vi "INV B - Current Sense Test.vi"(8 "error in (no error)":errorcluster, 10 "Message IN":string, 11 "Board Selector":T1) -> (0 "error out":errorcluster, 1 "Result (bool)":bool, 2 "Message OUT":string, 3 "VISA OUT":refnum<visa-resource-name>, 5 "Sense W":dbl, 7 "Sense V":dbl, 9 "Sense U":dbl)   [LabVIEW 2022 SP3]
uses:
  Serial Board Com/Board Select.ctl
  Serial Board Com/ADCSelector BB.ctl
  Serial Board Com/ADCSelector GB.ctl
  HMP4000 Communication/HMP4040_ChannelControl.ctl
panel:
  out "INVA_ISENSE_W":bool
  out "INVA_ISENSE_V":bool
  out "INVA_ISENSE_U":bool
  out "Result (color)":u32(colorbox)
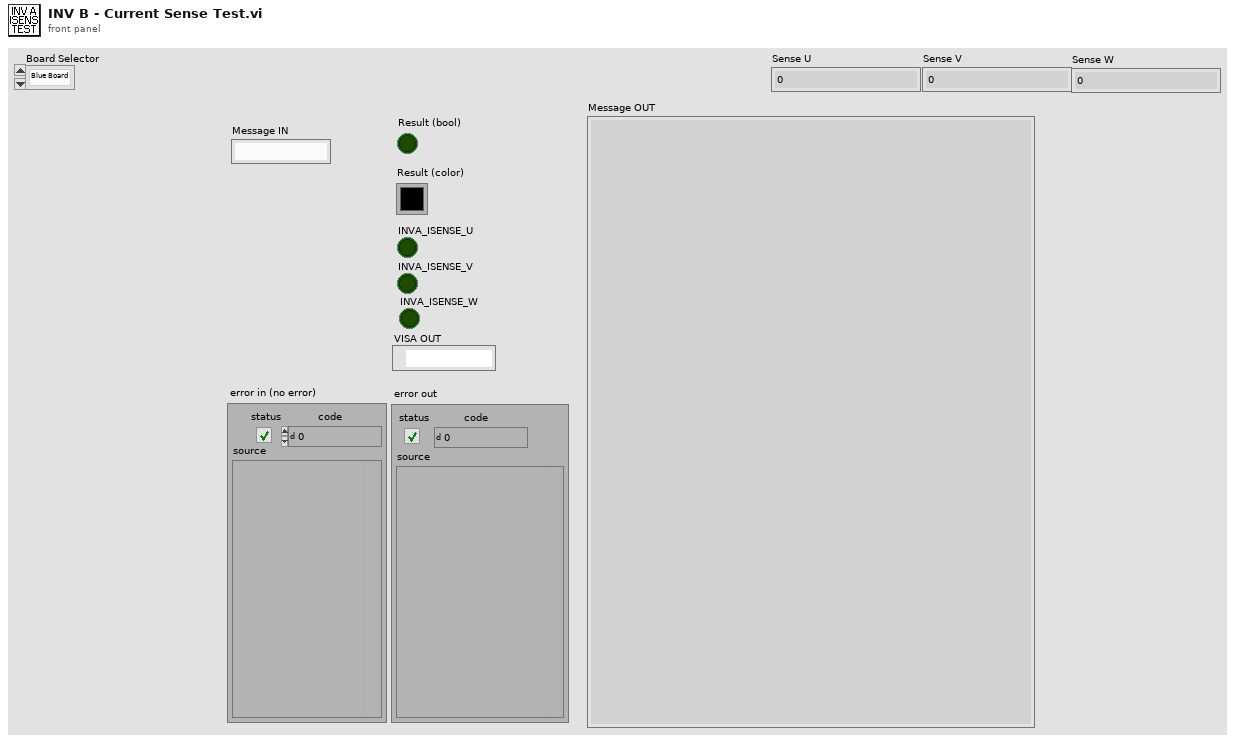
[diagram p1: front panel]
types:
  T1 = typedef "Board Select.ctl" = enum16{"Blue Board", "Green Board"}
  T2 = typedef "HMP4040_ChannelControl.ctl" = cluster{"CH1 Voltage":dbl, "CH1 Current":dbl, "CH1 Output":bool, "CH2 Voltage":dbl, "CH2 Current":dbl, "CH2 Output":bool, "CH3 Voltage":dbl, "CH3 Current":dbl, "CH3 Output":bool, "CH4 Voltage":dbl, "CH4 Current":dbl, "CH4 Output":bool, "Master Output":bool}
  T3 = typedef "ADCSelector GB.ctl" = enum16{"INVA_ISENSE_U", "INVA_ISENSE_V", "INVA_ISENSE_W", "INVA_UDC", "INVA_TEMP", "HB_ISENSE", "AUX_ISENSE_U", "AUX_ISENSE_V", "AUX_ISENSE_W", "VLINE_AB", "VLINE_BC", "VLINE_CA", "REF_1P5V", "VSENSE_POS_24V", "VSENSE_POS_5V", "VSENSE_NEG_15V", "TEST_POINT", "INVB_ISENSE_U", "INVB_ISENSE_V", "INVB_ISENSE_W", "INVB_UDC", "INVB_TEMP", "HB_TEMP", "AUXA_TEMP", "AUXB_TEMP", "AUXC_TEMP", "VOUT_AB", "VOUT_BC", "VOUT_CA", "REF_2P5V", "VSENSE_POS_15V", "VSENSE_POS_3P3V", "NET_ANALYZER"}
  T4 = typedef "ADCSelector BB.ctl" = enum16{"INVA_ISENSE_U", "INVA_ISENSE_V", "INVA_ISENSE_W", "INVA_UDC", "INVA_TEMP", "HB_TEMP", "AUXB_TEMP", "VLINE_AB", "VLINE_BC", "VLINE_CA", "VSENSE_POS_24V", "VSENSE_POS_5V", "VSENSE_NEG_15V", "INVB_ISENSE_U", "INV_B_ISENSEV", "INVB_ISENSE_W", "INVB_UDC", "INVB_TEMP", "AUXA_TEMP", "AUXC_TEMP", "VOUT_AB", "VOUT_BC", "VOUT_CA", "VSENSE_POS_15V", "VSENSE_POS_3P3V", "TEST_POINT"}
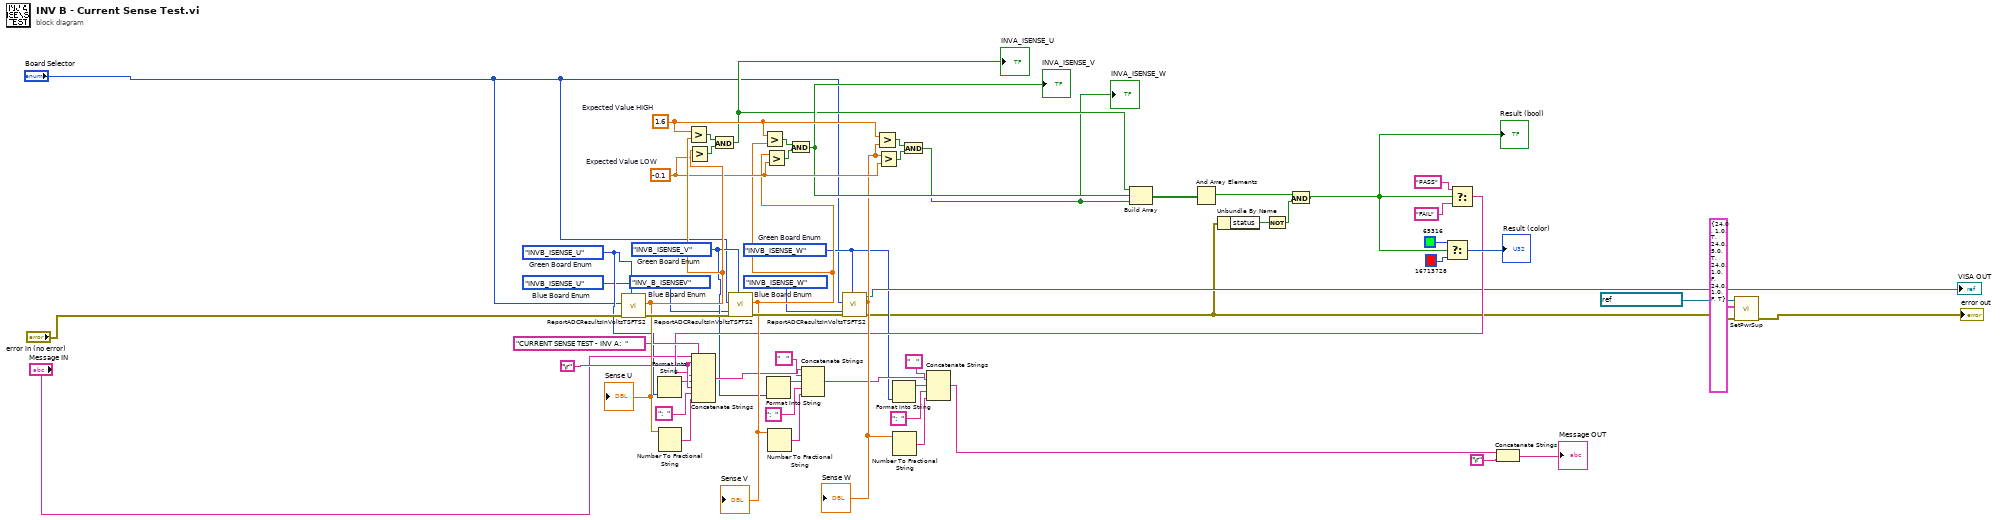
[diagram p0: block diagram]
diagram:
  w9 = ADCSelector_GB."INVB_ISENSE_W"  # Green Board Enum
  w10 = ADCSelector_GB."INVB_ISENSE_V"  # Green Board Enum
  w11 = ADCSelector_GB."INVB_ISENSE_U"  # Green Board Enum
  w16 = "\r"
  w33 = -0.1  # Expected Value LOW
  w32 = 1.6  # Expected Value HIGH
  w1 = ADCSelector_BB."INVB_ISENSE_W"  # Blue Board Enum
  w2 = ADCSelector_BB."INV_B_ISENSEV"  # Blue Board Enum
  w3 = ADCSelector_BB."INVB_ISENSE_U"  # Blue Board Enum
  n1 = call "ReportADCResultsInVoltsTSFTS2.vi"("Blue Board Enum"=w3, "Green Board Enum"=w11, "error in (no error)"="error in (no error)", "Board Selector"="Board Selector") -> ("error out"=w50:errorcluster, "Result"=w40:dbl)  [unwired: 4 in, 2 out]
  "Sense U" <- w40
  n2 = Format Into String(w11) -> (resulting string=w17:string)  [unwired: 3 in, 1 out]
  n3 = Number To Fractional String(number=w40) -> (F-format string=w19:string)  [unwired: 3 in]
  n4 = Greater?(x=w32, y=w40) -> (0:w39:bool)
  n5 = Greater?(x=w40, y=w33) -> (0:w38:bool)
  n6 = And(x=w39, y=w38) -> (x .and. y?=w30:bool)
  "INVA_ISENSE_U" <- w30
  n7 = call "ReportADCResultsInVoltsTSFTS2.vi"("Blue Board Enum"=w2, "Green Board Enum"=w10, "error in (no error)"=w50, "Board Selector"="Board Selector") -> ("error out"=w49:errorcluster, "Result"=w29:dbl)  [unwired: 4 in, 2 out]
  "Sense V" <- w29
  n8 = Greater?(x=w32, y=w29) -> (0:w36:bool)
  n9 = Greater?(x=w29, y=w33) -> (0:w37:bool)
  n10 = Format Into String(w10) -> (resulting string=w46:string)  [unwired: 3 in, 1 out]
  n11 = Number To Fractional String(number=w29) -> (F-format string=w47:string)  [unwired: 3 in]
  n12 = And(x=w36, y=w37) -> (x .and. y?=w31:bool)
  "INVA_ISENSE_V" <- w31
  n13 = call "ReportADCResultsInVoltsTSFTS2.vi"("Blue Board Enum"=w1, "Green Board Enum"=w9, "error in (no error)"=w49, "Board Selector"="Board Selector") -> ("error out"=w8:errorcluster, "Result"=w28:dbl, "VISA Refnum out"=→"VISA OUT":refnum<visa-resource-name>)  [unwired: 4 in, 1 out]
  "Sense W" <- w28
  n14 = Greater?(x=w32, y=w28) -> (0:w35:bool)
  n15 = Greater?(x=w28, y=w33) -> (0:w34:bool)
  n16 = Format Into String(w9) -> (resulting string=w45:string)  [unwired: 3 in, 1 out]
  n17 = Number To Fractional String(number=w28) -> (F-format string=w44:string)  [unwired: 3 in]
  n18 = And(x=w35, y=w34) -> (x .and. y?=w27:bool)
  "INVA_ISENSE_W" <- w27
  n19 = Build Array(w30, w31, w27) -> (w42:bool[])
  n20 = And Array Elements(Boolean array=w42) -> (logical AND=w53:bool)
  n21 = Unbundle By Name(w8) -> ("status"=w41:bool)
  n22 = Not(x=w41) -> (.not. x?=w52:bool)
  n23 = And(x=w53, y=w52) -> (x .and. y?=w54:bool)
  "Result (bool)" <- w54
  n24 = Select(t=u32 65316 ("Result (color)"), s=w54, f=u32 16713728 ("Result (color)")) -> (s? t:f=→"Result (color)":u32)
  n25 = Select(t="PASS", s=w54, f="FAIL") -> (s? t:f=w15:string)
  n26 = Concatenate Strings("Message IN", w16, "CURRENT SENSE TEST - INV A:  ", w15, w16, w17, ":  ", w19) -> (w26:string)
  n27 = Concatenate Strings(w26, "   ", w46, ":  ", w47) -> (w23:string)
  n28 = Concatenate Strings(w23, "   ", w45, ":  ", w44) -> (w22:string)
  n29 = Concatenate Strings(w22, "\r") -> (→"Message OUT":string)
  n30 = call "SetPwrSup.vi"("error in (no error)"=w8, "HMP4040 Channel Settings"=T2 {"CH1 Voltage"=24.0, "CH1 Current"=1.0, "CH1 Output"=TRUE, "CH2 Voltage"=24.0, "CH2 Current"=5.0, "CH2 Output"=TRUE, "CH3 Voltage"=24.0, "CH3 Current"=1.0, "CH3 Output"=FALSE, "CH4 Voltage"=24.0, "CH4 Current"=1.0, "CH4 Output"=FALSE, "Master Output"=TRUE}, "HMP4040 IN"=refnum<visa-resource-name> "HMP4040_FTS2" ("VISA resource name")) -> ("error out"=→"error out":errorcluster)  [unwired: 7 in, 1 out]
